vi "DAQ 카운터(펄스트레인, 에지카운트 측정).vi"() -> ()   [LabVIEW 2020]
uses:
  <vilib>/DAQmx/read.llb/DAQmx Read (Counter 1D U32 1Chan NSamp).vi
  <vilib>/DAQmx/create/channels.llb/DAQmx Create Channel (CO-Pulse Generation-Frequency).vi
  <vilib>/DAQmx/configure/timing.llb/DAQmx Timing (Implicit).vi
  <vilib>/DAQmx/create/channels.llb/DAQmx Create Channel (CI-Count Edges).vi
  <vilib>/DAQmx/configure/timing.llb/DAQmx Timing (Sample Clock).vi
  <vilib>/DAQmx/miscellaneous.llb/DAQmx Fill In Error Info.vi
panel:
  out "data":u32[](array[numeric]) caption="데이터"
  in  "정지":bool
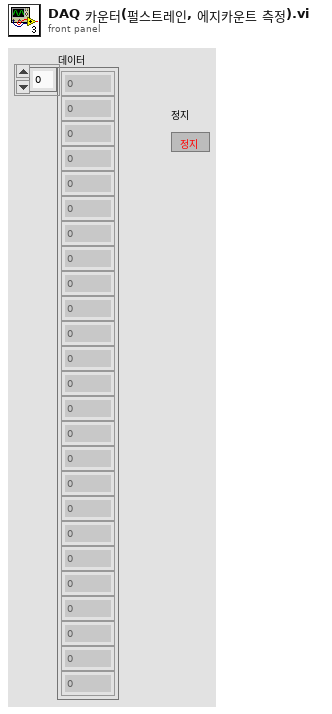
[diagram p1: front panel]
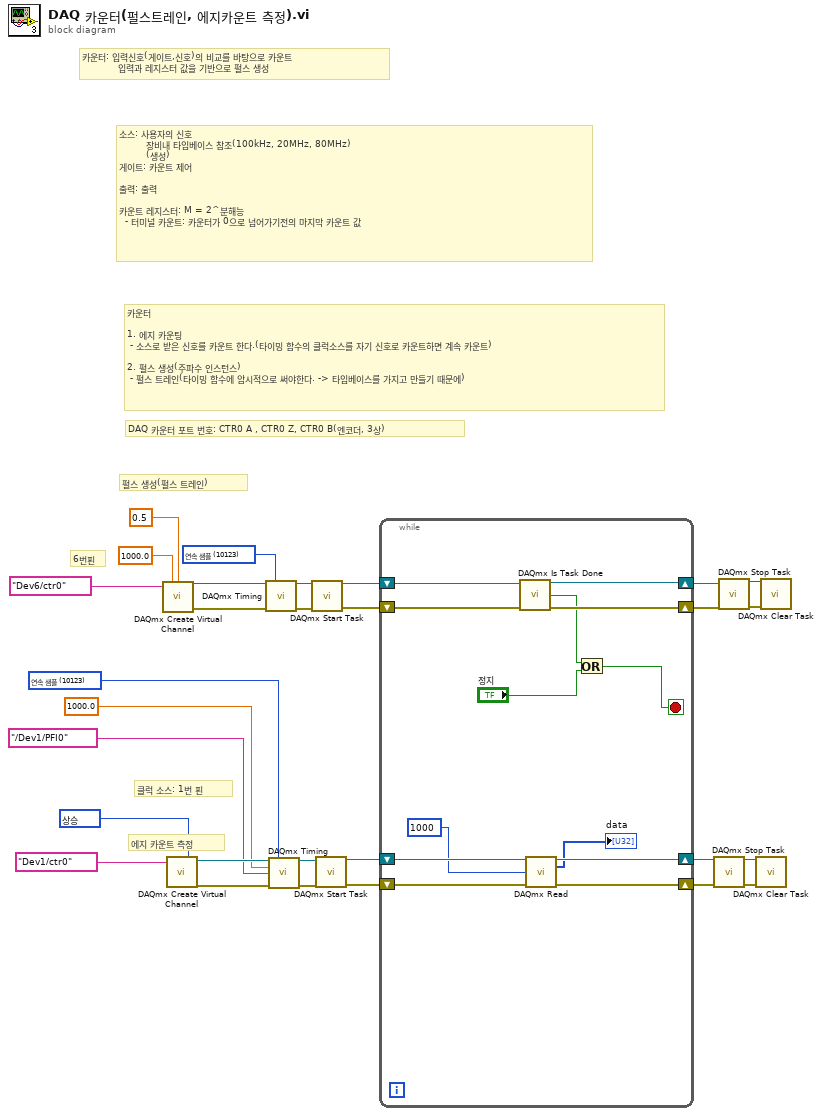
[diagram p0: block diagram]
diagram:
  w9 = 10123 items=["유한 샘플"=10178, "연속 샘플"=10123, "하드웨어 타이밍에 의한 단일 포인트"=12522] ("sample mode")
  w15 = 10280 items=["상승"=10280, "하강"=10171] ("edge")
  w26 = 10123 items=["유한 샘플"=10178, "연속 샘플"=10123, "하드웨어 타이밍에 의한 단일 포인트"=12522] ("sample mode")
  # "에지 카운트 측정"
  # "클럭 소스: 1번 핀"
  # "펄스 생성(펄스 트레인)"
  # "6번핀"
  # "DAQ 카운터 포트 번호: CTR0 A , CTR0 Z, CTR0 B(엔코더, 3상)"
  # "카운터\n\n1. 에지 카운팅\n - 소스로 받은 신호를 카운트 한다.(타이밍 함수의 클럭소스를 자기 신호로 카운트하면 계속 카운트)\n \n2. 펄스 생성(주파수 인스턴스)\n - 펄스 트레인(타이밍 함수에 암시적으로 써야한다. -> 타임베이스를 가지고 만들기 때문에)"
  # "소스: 사용자의 신호\n         장비내 타임베이스 참조(100kHz, 20MHz, 80MHz)\n         (생성)\n게이트: 카운트 제어\n\n출력: 출력\n\n카운트 레지스터: M = 2^분해능\n  - 터미널 카운트: 카운터가 0으로 넘어가기전의 마지막 카운트 값"
  # "카운터: 입력신호(게이트,신호)의 비교를 바탕으로 카운트\n            입력과 레지스터 값을 기반으로 펄스 생성"
  n1 = call-poly <vilib>:"DAQmx Create Virtual Channel.vi"("frequency"=1000.0, "duty cycle"=0.5, "counter"=tag "Dev6/ctr0") -> ("task out"=w28:refnum<k21>, "error out"=w27:errorcluster)  [unwired: 11 in]
  n2 = call-poly <vilib>:"DAQmx Create Virtual Channel.vi"("edge"=w15, "counter"=tag "Dev1/ctr0") -> ("task out"=w13:refnum<k21>, "error out"=w12:errorcluster)  [unwired: 12 in]
  n3 = call-poly <vilib>:"DAQmx Timing.vi"("task/channels in"=w28, "sample mode"=w26, "error in"=w27) -> ("task out"=w23:refnum<k21>, "error out"=w22:errorcluster)  [unwired: 11 in]
  n4 = call-poly <vilib>:"DAQmx Timing.vi"("task/channels in"=w13, "sample mode"=w9, "rate"=1000.0, "source"=tag "/Dev1/PFI0", "error in"=w12) -> ("task out"=w8:refnum<k21>, "error out"=w7:errorcluster)  [unwired: 9 in]
  n5 = call <vilib>:"DAQmx Start Task.vi"("task/channels in"=w23, "error in"=w22) -> ("task out"=w21:refnum<k21>, "error out"=w20:errorcluster)  [unwired: 12 in]
  n6 = call <vilib>:"DAQmx Start Task.vi"("task/channels in"=w8, "error in"=w7) -> ("task out"=w6:refnum<k21>, "error out"=w5:errorcluster)  [unwired: 12 in]
  n7 = while {
    shift-right: [w40] -> w19
    shift-left: w21 -> [w42]
    shift-right: [w39] -> w18
    shift-left: w20 -> [w41]
    shift-right: [w32] -> w2
    shift-left: w6 -> [w35]
    shift-right: [w31] -> w1
    shift-left: w5 -> [w34]
    stop <- w36 stop-if-true
    n8 = call <vilib>:"DAQmx Is Task Done.vi"("task/channels in"=w42, "error in"=w41) -> ("task out"=w40:refnum<k21>, "task done?"=w38:bool, "error out"=w39:errorcluster)  [unwired: 11 in]
    n9 = call-poly <vilib>:"DAQmx Read.vi"("task/channels in"=w35, "number of samples per channel"=1000, "error in"=w34) -> ("task out"=w32:refnum<k21>, "data"=→"data":u32[], "error out"=w31:errorcluster)  [unwired: 10 in]
    n10 = Or(x=w38, y="정지") -> (x .or. y?=w36:bool)
  }
  n11 = call <vilib>:"DAQmx Stop Task.vi"("task/channels in"=w2, "error in"=w1) -> ("task out"=w3:refnum<k21>, "error out"=w4:errorcluster)  [unwired: 12 in]
  n12 = call <vilib>:"DAQmx Stop Task.vi"("task/channels in"=w19, "error in"=w18) -> ("task out"=w17:refnum<k21>, "error out"=w16:errorcluster)  [unwired: 12 in]
  n13 = call <vilib>:"DAQmx Clear Task.vi"("task in"=w3, "error in"=w4) -> ()  [unwired: 13 in, 1 out]
  n14 = call <vilib>:"DAQmx Clear Task.vi"("task in"=w17, "error in"=w16) -> ()  [unwired: 13 in, 1 out]
